vi "generate_DAC_voltages.vi"(8 "derived values":T1, 9 "scan specification":T4={"x amplitude"=0, "x resolution (pixels)"=0, "x offset fly-forward (iterations)"=0, "x offset fly-back (iterations)"=0, "y resolution (nr. of lines)"=0, "y step size"=0, "iterations per pixel"=0, "number of frames"=0, "y offset (pixels)"=0, "number of y-brake lines  (before y-fly-back)"=0, "number y-brake lines (after y-fly-back)"=0, "y-fly-back step size"=8, "number of y-fly-back steps"=0}, 10 "counter cluster in":T2, 11 "resonant trigger":bool) -> (0 "acquire?":bool, 1 "fly-back acquisition phase?":bool, 2 "counter cluster out":T2, 3 "DAC voltages":T3 {"ch6" max=4095 step=1; "ch5" max=4095 step=1; "ch4" max=4095 step=1; "ch3" max=4095 step=1; "ch2" max=4095 step=1; "ch1" max=4095 step=1; "ch0" max=4095 step=1})   [LabVIEW 2010]
uses:
  scan_specification_cluster.ctl
  common_typedefs/DAC_voltage_cluster.ctl
  counter_cluster.ctl
  derived_values_cluster.ctl
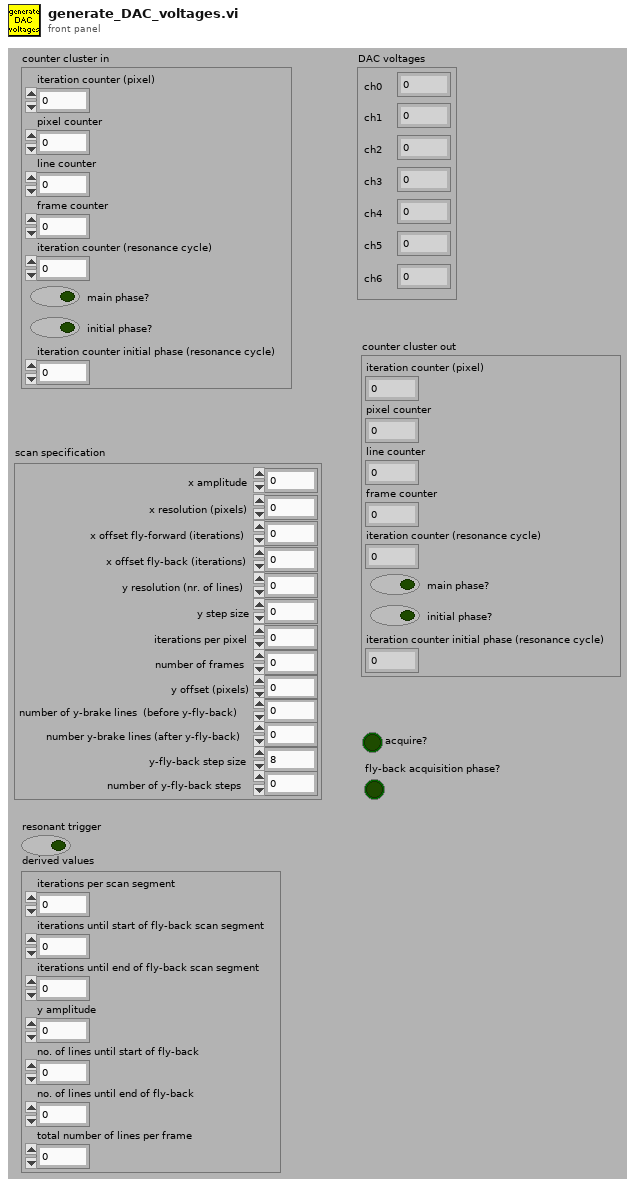
[diagram p1: front panel]
types:
  T1 = typedef "derived_values_cluster.ctl" = cluster{"iterations per scan segment":u16, "iterations until start of fly-back scan segment":u16, "iterations until end of fly-back scan segment":u16, "y amplitude":u16, "no. of lines until start of fly-back":u16, "no. of lines until end of fly-back":u16, "total number of lines per frame ":u16}
  T2 = typedef "counter_cluster.ctl" = cluster{"iteration counter (pixel)":u16, "pixel counter":u16, "line counter":u16, "frame counter":u16, "iteration counter (resonance cycle)":u16, "main phase?":bool, "initial phase?":bool, "iteration counter initial phase (resonance cycle)":u16}
  T3 = typedef "DAC_voltage_cluster.ctl" = cluster{"ch0":u16, "ch1":u16, "ch2":u16, "ch3":u16, "ch4":u16, "ch5":u16, "ch6":u16}
  T4 = typedef "scan_specification_cluster.ctl" = cluster{"x amplitude":u16, "x resolution (pixels)":u16, "x offset fly-forward (iterations)":u16, "x offset fly-back (iterations)":u16, "y resolution (nr. of lines)":u16, "y step size":u16, "iterations per pixel":u16, "number of frames":i32, "y offset (pixels)":u16, "number of y-brake lines  (before y-fly-back)":u16, "number y-brake lines (after y-fly-back)":u16, "y-fly-back step size":u16, "number of y-fly-back steps":u16}
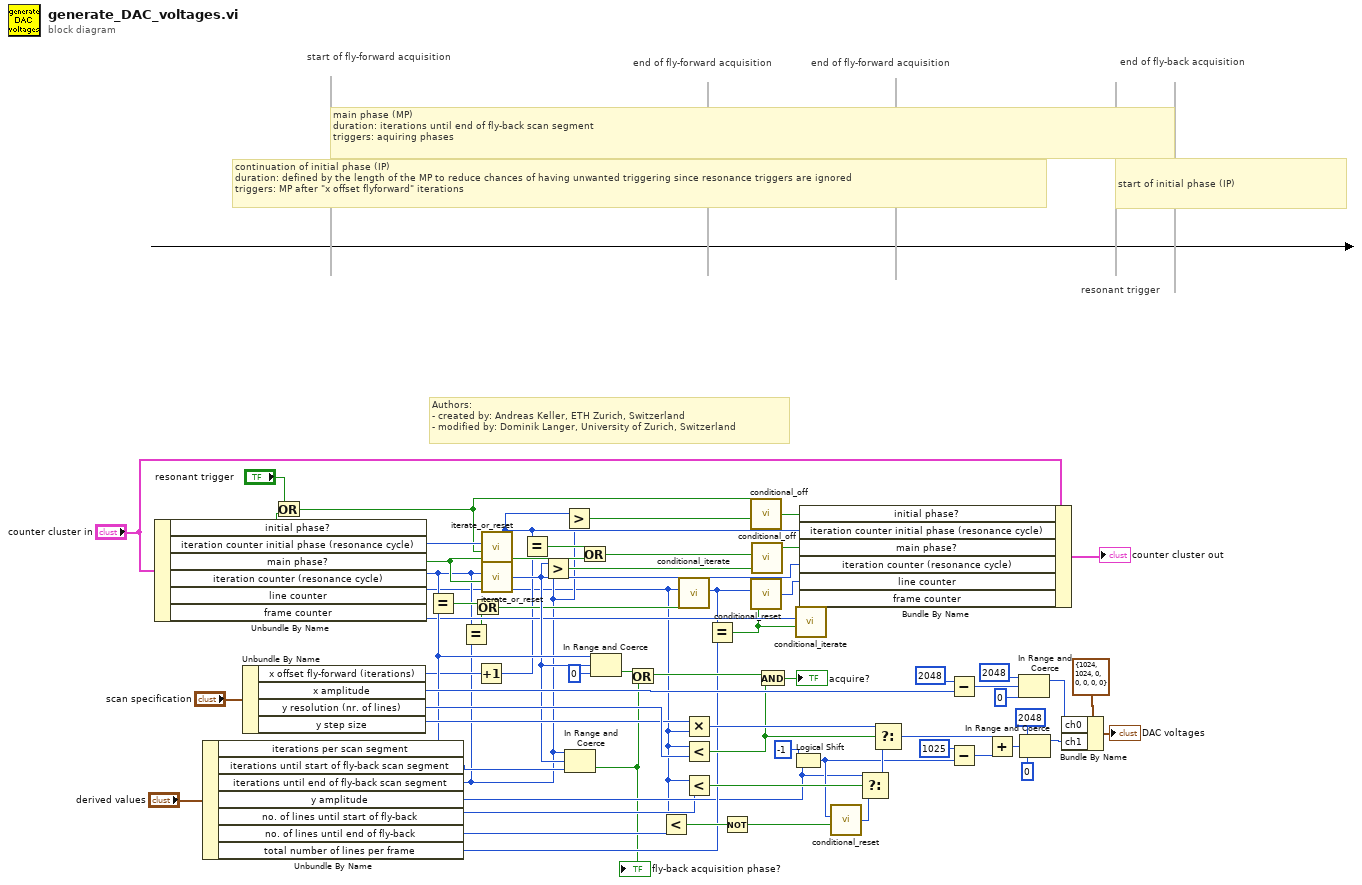
[diagram p0: block diagram]
diagram:
  # "start of initial phase (IP)"
  # "continuation of initial phase (IP)\nduration: defined by the length of the MP to reduce chances of having unwanted triggering since resonance triggers are ignored\ntriggers: MP after \"x offset flyforward\" iterations"
  # "end of fly-back acquisition"
  # "end of fly-forward acquisition"
  # "end of fly-forward acquisition"
  # "start of fly-forward acquisition"
  # "main phase (MP)\nduration: iterations until end of fly-back scan segment\ntriggers: aquiring phases"
  # "resonant trigger"
  # "Authors: \n- created by: Andreas Keller, ETH Zurich, Switzerland\n- modified by: Dominik Langer, University of Zurich, Switzerland"
  n1 = Unbundle By Name("counter cluster in") -> ("initial phase?"=w35:bool, "iteration counter initial phase (resonance cycle)"=w29:u16, "main phase?"=w28:bool, "iteration counter (resonance cycle)"=w6:u16, "line counter"=w3:u16, "frame counter"=w26:u16)
  n2 = Unbundle By Name("derived values") -> ("iterations per scan segment"=w32:u16, "iterations until start of fly-back scan segment"=w37:u16, "iterations until end of fly-back scan segment"=w5:u16, "y amplitude"=w14:u16, "no. of lines until start of fly-back"=w13:u16, "no. of lines until end of fly-back"=w36:u16, "total number of lines per frame"=w33:u16)
  n3 = Unbundle By Name("scan specification") -> ("x offset fly-forward (iterations)"=w11:u16, "x amplitude"=w46:u16, "y resolution (nr. of lines)"=w43:u16, "y step size"=w42:u16)
  n4 = Or(x="resonant trigger", y=w35) -> (x .or. y?=w22:bool)
  n5 = Equal?(x=w6, y=w32) -> (x = y?=w7:bool)
  n6 = Equal?(x=w6, y=w5) -> (x = y?=w4:bool)
  n7 = Or(x=w7, y=w4) -> (x .or. y?=w24:bool)
  n8 = Increment(x=w11) -> (x+1=w10:u16)
  n9 = call "iterate_or_reset.vi"("iterate?"=w22, "number in"=w29) -> ("number out"=w8:u16)  [unwired: 4 in]
  n10 = call "iterate_or_reset.vi"("iterate?"=w28, "number in"=w6) -> ("number out"=w27:u16)  [unwired: 4 in]
  n11 = Equal?(x=w8, y=w10) -> (x = y?=w23:bool)
  n12 = Greater?(x=w27, y=w5) -> (0:w20:bool)
  n13 = Greater?(x=w8, y=w5) -> (0:w9:bool)
  n14 = In Range and Coerce(upper limit=w5, x=w27, lower limit=w37) -> (In Range?=w1:bool)  [unwired: 1 out]
  "fly-back acquisition phase?" <- w1
  n15 = Or(x=w23, y=w28) -> (x .or. y?=w19:bool)
  n16 = In Range and Coerce(upper limit=w32, x=w27, lower limit=u16 0) -> (In Range?=w58:bool)  [unwired: 1 out]
  n17 = Or(x=w58, y=w1) -> (x .or. y?=w41:bool)
  n18 = Less?(x=w3, y=w36) -> (x < y?=w39:bool)
  n19 = call "conditional_iterate.vi"("iterate?"=w24, "number in"=w3) -> ("number out"=w2:u16)  [unwired: 4 in]
  n20 = Multiply(x=w42, y=w3) -> (x*y=w64:u16)
  n21 = Less?(x=w3, y=w43) -> (x < y?=w40:bool)
  n22 = Less?(x=w3, y=w13) -> (x < y?=w66:bool)
  n23 = Equal?(x=w2, y=w33) -> (x = y?=w12:bool)
  n24 = Not(x=w39) -> (.not. x?=w16:bool)
  n25 = call "conditional_off.vi"("switch off?"=w9, "boolean in"=w22) -> ("boolean out"=w21:bool)  [unwired: 4 in]
  n26 = call "conditional_reset.vi"("reset?"=w12, "number in"=w2) -> ("number out"=w30:u16)  [unwired: 4 in]
  n27 = call "conditional_off.vi"("switch off?"=w20, "boolean in"=w19) -> ("boolean out"=w18:bool)  [unwired: 4 in]
  n28 = And(x=w41, y=w40) -> (x .and. y?=→"acquire?":bool)
  n29 = Logical Shift(y=i16 -1 ("n"), x=w14) -> (x << y=w17:u16)
  n30 = call "conditional_iterate.vi"("iterate?"=w12, "number in"=w26) -> ("number out"=w25:u16)  [unwired: 4 in]
  n31 = Bundle By Name(cluster="counter cluster in", "initial phase?"=w21, "iteration counter initial phase (resonance cycle)"=w8, "main phase?"=w18, "iteration counter (resonance cycle)"=w27, "line counter"=w30, "frame counter"=w25) -> (→"counter cluster out":T2)
  n32 = call "conditional_reset.vi"("reset?"=w16, "number in"=w17) -> ("number out"=w15:u16)  [unwired: 4 in]
  n33 = Select(t=w14, s=w66, f=w15) -> (s? t:f=w65:u16)
  n34 = Select(t=w64, s=w40, f=w65) -> (s? t:f=w44:u16)
  n35 = Subtract(x=u16 2048, y=w46) -> (x-y=w50:u16)
  n36 = Subtract(x=u16 1025, y=w17) -> (x-y=w57:u16)
  n37 = Add(x=w44, y=w57) -> (x+y=w53:u16)
  n38 = In Range and Coerce(upper limit=u16 2048, x=w50, lower limit=u16 0) -> (coerced(x)=w49:u16)  [unwired: 1 out]
  n39 = In Range and Coerce(upper limit=u16 2048, x=w53, lower limit=u16 0) -> (coerced(x)=w52:u16)  [unwired: 1 out]
  n40 = Bundle By Name(cluster=T3 {"ch0"=1024, "ch1"=1024, "ch2"=0, "ch3"=0, "ch4"=0, "ch5"=0, "ch6"=0} ("DAC voltage"), "ch0"=w49, "ch1"=w52) -> (→"DAC voltages":T3)
